vi "Error Log.vi"(8 "error in (no error)":errorcluster) -> (0 "error out":errorcluster)   [LabVIEW 2017]
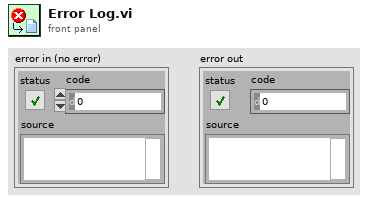
[diagram p1: front panel]
types:
  T1 = enum16{"open", "replace", "create", "open or create", "replace or create", "replace or create with confirmation"}
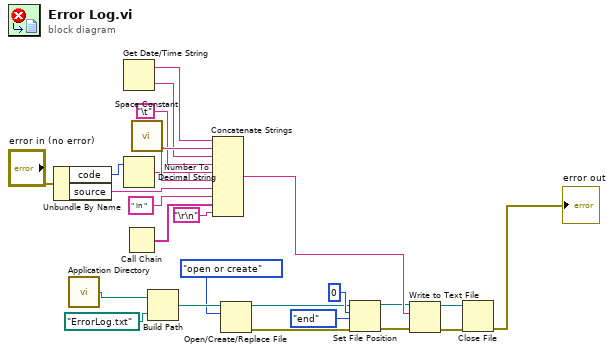
[diagram p0: block diagram]
diagram:
  n1 = Unbundle By Name("error in (no error)") -> ("code"=w5:i32, "source"=w8:string)
  n2 = call <vilib>:"Application Directory.vi"() -> ("Application Directory"=w14:path)
  n3 = Get Date/Time String() -> (date string=w2:string, time string=w3:string)  [unwired: 3 in]
  n4 = Number To Decimal String(number=w5) -> (decimal integer string=w6:string)  [unwired: 1 in]
  n5 = Call Chain() -> (call chain=w10:string[])
  n6 = call <vilib>:"Space Constant.vi"() -> ("String"=w7:string)
  n7 = Build Path(base path=w14, name or relative path=path "ErrorLog.txt") -> (appended path=w15:path)
  n8 = Concatenate Strings(w2, w7, w3, "\t", w6, w7, w8, " in " ("string"), w10, "\r\n") -> (w25:string)
  n9 = Open/Create/Replace File(file path (use dialog)=w15, operation (0:open)=T1."open or create") -> (refnum out=w19:refnum<file>, error out=w22:errorcluster)  [unwired: 4 in, 1 out]
  n10 = Set File Position(offset (in bytes) (0)=i64 0, refnum=w19, from (0:start)=enum16{"start", "end", "current"}."end", error in=w22) -> (refnum out=w20:refnum<file>, error out=w21:errorcluster)
  n11 = Write to Text File(file (use dialog)=w20, text=w25, error in=w21) -> (refnum out=w17:refnum<file>, error out=w16:errorcluster)  [unwired: 1 in, 1 out]
  n12 = Close File(refnum=w17, error in=w16) -> (error out=→"error out":errorcluster)  [unwired: 1 out]
